vi "main -2.0.vi"() -> ()   [LabVIEW 2018]
uses:
  <vilib>/Analysis/baseanly.llb/Mean (DBL).vi
  <vilib>/Instr/_visa.llb/VISA Configure Serial Port (Instr).vi
  <vilib>/Analysis/NI_AALBase.lvlib
panel:
  out "十六进制整型字符串":string
  out "提示":string
  out "错误指示":bool
  in  "单片机COM":refnum<visa-resource-name>
  out "上一路数据图":dbl[](graph)
  in  "数据存储位置":path
  in  "开关":bool
  out "2-7 2":bool
  out "2-6 2":bool
  out "2-5 2":bool
  out "2-4 2":bool
  out "2-3 2":bool
  out "2-2 2":bool
  out "2-1 2":bool
  out "1-7 2":bool
  out "1-6 2":bool
  out "1-5 2":bool
  out "1-4 2":bool
  out "1-3 2":bool
  out "1-2 2":bool
  out "1-1 2":bool
  out "字符串":string
  in  "1-7":bool
  in  "2-7":bool
  in  "2-6":bool
  in  "2-5":bool
  in  "2-4":bool
  in  "2-3":bool
  in  "2-2":bool
  in  "2-1":bool
  in  "1-1":bool
  in  "1-2":bool
  in  "1-3":bool
  in  "1-4":bool
  in  "1-5":bool
  in  "1-6":bool
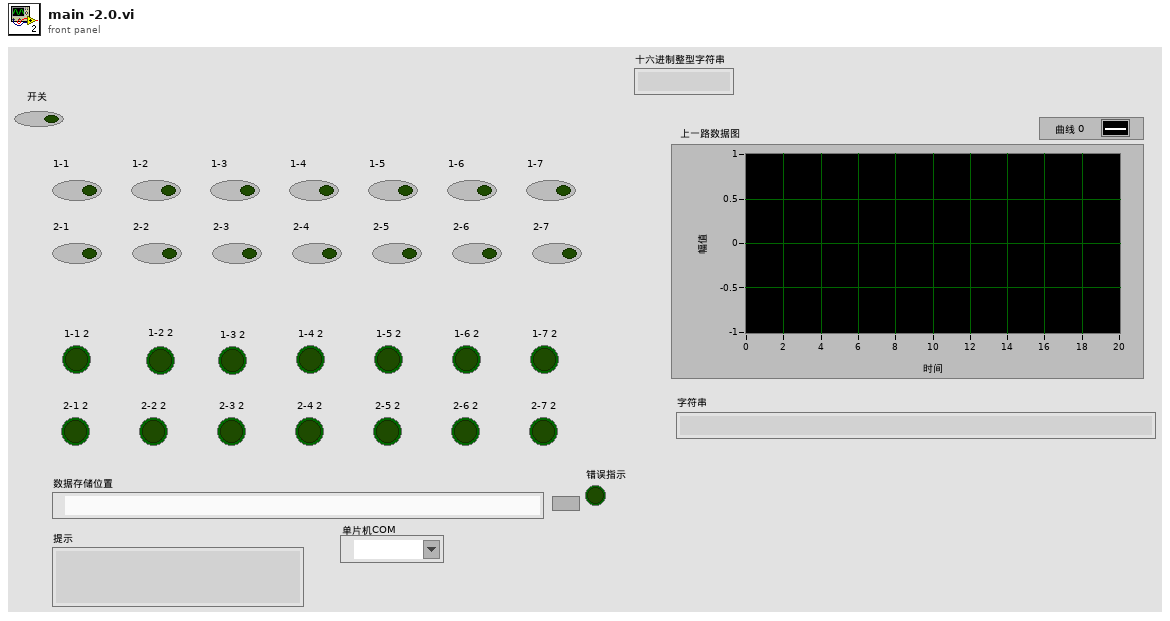
[diagram p1: front panel]
types:
  T1 = enum16{"open", "replace", "create", "open or create", "replace or create", "replace or create with confirmation"}
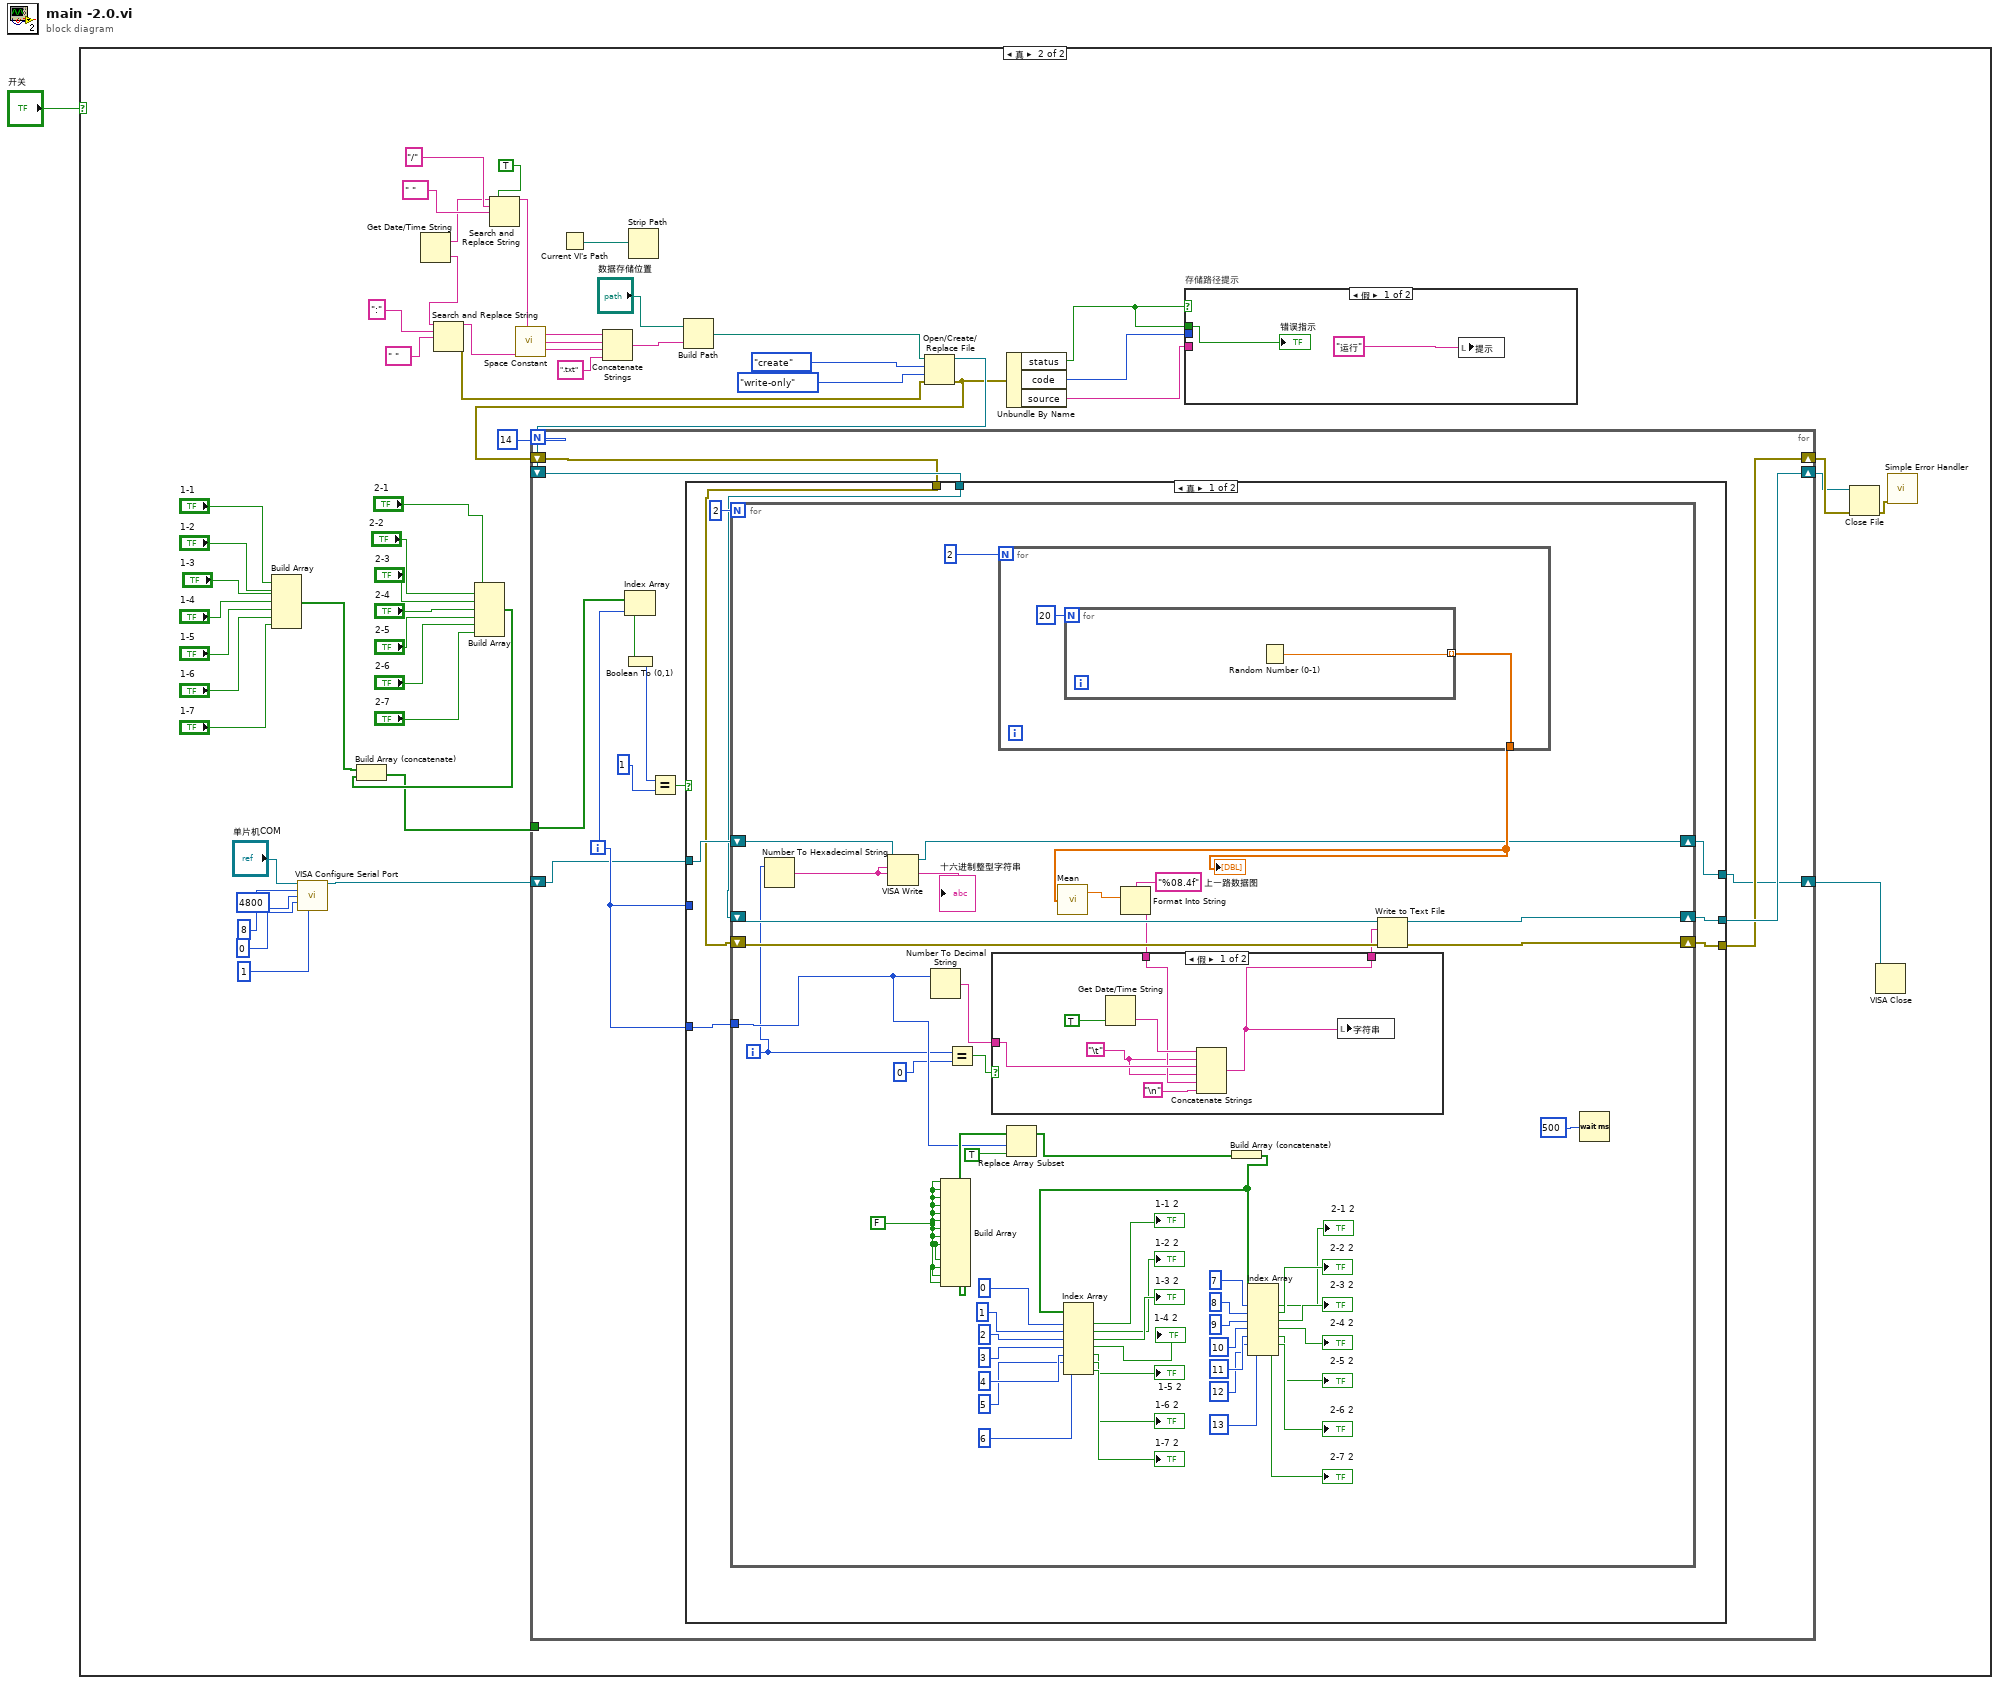
[diagram p0: block diagram]
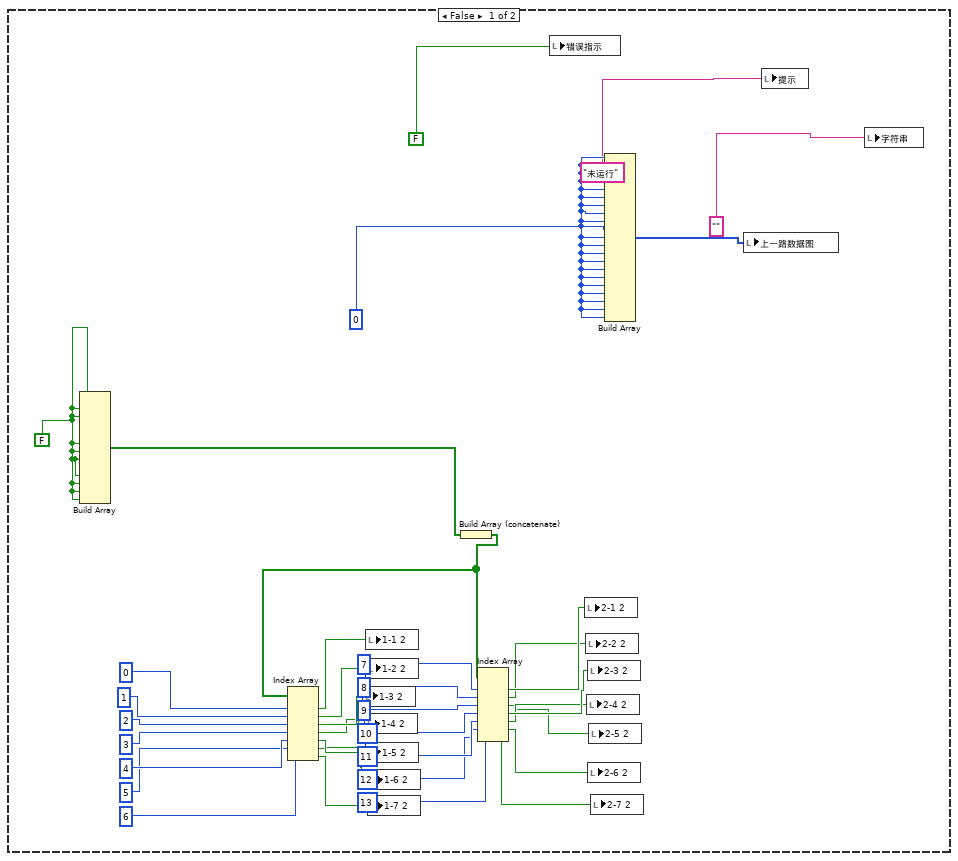
[diagram p2: hidden frame]
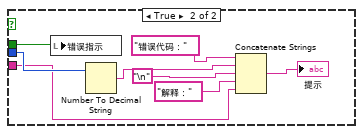
[diagram p3: hidden frame]
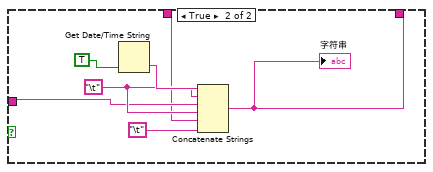
[diagram p4: hidden frame]
diagram:
  n1 = case shown="真" "开关" {
    frame False {
      w5 = 0
      w37 = FALSE
      n2 = Build Array(w37, w37, w37, w37, w37, w37, w37, w37, w37, w37, w37, w37, w37, w37) -> (w21:bool[])
      n3 = Build Array (concatenate)(w21) -> (w36:bool[])
      n4 = Index Array(array=w36, index #1=0, index #2=1, index #3=2, index #4=3, index #5=4, index #6=5, index #7=6) -> (element #1=w13:bool, element #2=w12:bool, element #3=w11:bool, element #4=w10:bool, element #5=w9:bool, element #6=w8:bool, element #7=w7:bool)
      n5 = local write "1-3 2"(w11) -> ()
      n6 = local write "1-4 2"(w10) -> ()
      n7 = local write "1-1 2"(w13) -> ()
      n8 = local write "1-2 2"(w12) -> ()
      n9 = local write "1-5 2"(w9) -> ()
      n10 = local write "1-6 2"(w8) -> ()
      n11 = local write "1-7 2"(w7) -> ()
      n12 = Index Array(array=w36, index #1=7, index #2=8, index #3=9, index #4=10, index #5=11, index #6=12, index #7=13) -> (element #1=w20:bool, element #2=w19:bool, element #3=w16:bool, element #4=w18:bool, element #5=w17:bool, element #6=w15:bool, element #7=w14:bool)
      n13 = local write "错误指示"(FALSE) -> ()
      n14 = local write "2-1 2"(w20) -> ()
      n15 = local write "2-2 2"(w19) -> ()
      n16 = local write "2-4 2"(w17) -> ()
      n17 = local write "2-3 2"(w18) -> ()
      n18 = local write "2-6 2"(w15) -> ()
      n19 = local write "2-5 2"(w16) -> ()
      n20 = local write "2-7 2"(w14) -> ()
      n21 = Build Array(w5, w5, w5, w5, w5, w5, w5, w5, w5, w5, w5, w5, w5, w5, w5, w5, w5, w5, w5, w5, w5) -> (w6:i32[])
      n22 = local write "上一路数据图"(w6) -> ()
      n23 = local write "提示"("未运行") -> ()
      n24 = local write "字符串"("") -> ()
    }
    frame True {
      n25 = Build Array("1-1", "1-2", "1-3", "1-4", "1-5", "1-6", "1-7") -> (w74:bool[])
      n26 = call-poly "VISA Configure Serial Port"("VISA resource name"="单片机COM", "baud rate (9600)"=4800, "data bits (8)"=8, "parity (0:none)"=0, "stop bits (10: 1 bit)"=1) -> ("VISA resource name out"=w42:refnum<visa-resource-name>)  [unwired: 9 in, 1 out]
      n27 = Get Date/Time String() -> (date string=w56:string, time string=w63:string)  [unwired: 3 in]
      n28 = Search and Replace String(input string=w63, search string=":", replace string=" ") -> (result string=w53:string, error out=w60:errorcluster)  [unwired: 5 in, 2 out]
      n29 = Build Array("2-1", "2-2", "2-3", "2-4", "2-5", "2-6", "2-7") -> (w73:bool[])
      n30 = Build Array (concatenate)(w74, w73) -> (w72:bool[])
      n31 = Search and Replace String(replace all?=TRUE, input string=w56, search string="/", replace string=" ") -> (result string=w55:string)  [unwired: 4 in, 3 out]
      n32 = call <vilib>:"Space Constant.vi"() -> ("String"=w59:string)
      n33 = Current VI's Path() -> (path=w66:path)
      n34 = Concatenate Strings(w55, w59, w53, ".txt") -> (w70:string)
      n35 = Strip Path(path=w66) -> ()  [unwired: 2 out]
      n36 = Build Path(base path="数据存储位置", name or relative path=w70) -> (appended path=w65:path)
      n37 = Open/Create/Replace File(file path (use dialog)=w65, error in=w60, operation (0:open)=T1."create", access (0:read/write)=enum16{"read/write", "read-only", "write-only"}."write-only") -> (refnum out=w67:refnum<file>, error out=w41:errorcluster)  [unwired: 3 out]
      n38 = for {
        N: 14 -> [_]
        tunnel: w72 -> [w102]
        shift-right: [w106] -> w51
        shift-left: w67 -> [w104]
        shift-right: [w105] -> w52
        shift-left: w41 -> [w103]
        shift-right: [w99] -> w43
        shift-left: w42 -> [w100]
        i -> [w101]
        n39 = Index Array(array=w102, index=w101) -> (element=w110:bool)
        n40 = Boolean To (0,1)(Boolean=w110) -> (0, 1=w108:i16)
        n41 = Equal?(x=w108, y=1) -> (x = y?=w107:bool)
        n42 = case shown="真" w107 {
          tunnel: w104 -> [w111 w189]
          tunnel: w101 -> [w116 _]
          tunnel: [w118 w189] -> w106
          tunnel: [w117 w190] -> w105
          tunnel: w103 -> [w112 w190]
          tunnel: w100 -> [w114 w188]
          tunnel: w101 -> [_ _]
          tunnel: [w113 w188] -> w99
          frame True {
            n43 = for {
              N: 2 -> [_]
              tunnel: w116 -> [w126]
              shift-right: [w169] -> w118
              shift-left: w111 -> [w170]
              shift-right: [w132] -> w117
              shift-left: w112 -> [w168]
              shift-right: [w121] -> w113
              shift-left: w114 -> [w122]
              i -> [w120]
              w165 = FALSE
              n44 = Number To Hexadecimal String(2:w120) -> (0:w119:string)  [unwired: 1 in]
              "十六进制整型字符串" <- w119
              n45 = VISA Write(VISA resource name=w122, write buffer=w119) -> (VISA resource name out=w121:refnum<visa-resource-name>)  [unwired: 1 in, 2 out]
              n46 = Number To Decimal String(number=w126) -> (decimal integer string=w167:string)  [unwired: 1 in]
              n47 = Build Array(w165, w165, w165, w165, w165, w165, w165, w165, w165, w165, w165, w165, w165, w165) -> (w164:bool[])
              n48 = Equal?(x=w120, y=0) -> (x = y?=w124:bool)
              n49 = for {
                N: 2 -> [_]
                tunnel: [w186] -> w128
                n50 = for {
                  N: 20 -> [_]
                  tunnel: [w187] -> w186 mode=indexing
                  n51 = Random Number (0-1)() -> (number: 0 to 1=w187:dbl)
                }
              }
              "上一路数据图" <- w128
              n52 = Replace Array Subset(array=w164, new element=TRUE, index=w126) -> (w133:bool[])
              n53 = call-poly <vilib>:"Mean.vi"("X"=w128) -> ("mean"=w130:dbl)  [unwired: 1 out]
              n54 = Format Into String(format string="%08.4f" ("格式字符串"), w130) -> (resulting string=w129:string)  [unwired: 2 in, 1 out]
              n55 = case shown="假" w124 {
                tunnel: w167 -> [w174 w181]
                tunnel: [w171 w180] -> w166
                tunnel: w129 -> [w173 w179]
                frame False {
                  w172 = "\t" ("Tab")
                  n56 = Get Date/Time String(want seconds? (F)=TRUE) -> (time string=w176:string)  [unwired: 2 in, 1 out]
                  n57 = Concatenate Strings(w176, w172, w174, w172, w173, "\n") -> (w171:string)
                  n58 = local write "字符串"(w171) -> ()
                }
                frame True {
                  w182 = "\t" ("Tab")
                  n59 = Get Date/Time String(want seconds? (F)=TRUE) -> (time string=w183:string)  [unwired: 2 in, 1 out]
                  n60 = Concatenate Strings(w183, w182, w181, w182, w179, "\t") -> (w180:string)
                  "字符串" <- w180
                }
              }
              n61 = Build Array (concatenate)(w133) -> (w148:bool[])
              n62 = Index Array(array=w148, index #1=0, index #2=1, index #3=2, index #4=3, index #5=4, index #6=5, index #7=6) -> (element #1=→"1-1 2":bool, element #2=→"1-2 2":bool, element #3=→"1-3 2":bool, element #4=→"1-4 2":bool, element #5=→"1-5 2":bool, element #6=→"1-6 2":bool, element #7=→"1-7 2":bool)
              n63 = Index Array(array=w148, index #1=7, index #2=8, index #3=9, index #4=10, index #5=11, index #6=12, index #7=13) -> (element #1=→"2-1 2":bool, element #2=→"2-2 2":bool, element #3=→"2-3 2":bool, element #4=→"2-4 2":bool, element #5=→"2-5 2":bool, element #6=→"2-6 2":bool, element #7=→"2-7 2":bool)
              n64 = Write to Text File(file (use dialog)=w170, text=w166, error in=w168) -> (refnum out=w169:refnum<file>, error out=w132:errorcluster)  [unwired: 1 in, 1 out]
              n65 = Wait (ms)(milliseconds to wait=u32 500) -> ()  [unwired: 1 out]
            }
          }
          frame False {
          }
        }
      }
      n66 = Unbundle By Name(w41) -> ("status"=w38:bool, "code"=w40:i32, "source"=w39:string)
      n67 = case "存储路径提示" shown="假" w38 {
        tunnel: w40 -> [_ w97]
        tunnel: w39 -> [_ w92]
        tunnel: w38 -> [w90 w98]
        frame False {
          n68 = local write "提示"("运行") -> ()
          "错误指示" <- w90
        }
        frame True {
          n69 = local write "错误指示"(w98) -> ()
          n70 = Number To Decimal String(number=w97) -> (decimal integer string=w95:string)  [unwired: 1 in]
          n71 = Concatenate Strings("错误代码：", w95, "\n", "解释：", w92) -> (→"提示":string)
        }
      }
      n72 = Close File(refnum=w51, error in=w52) -> (error out=w50:errorcluster)  [unwired: 1 out]
      n73 = VISA Close(VISA resource name=w43) -> ()  [unwired: 1 in, 1 out]
      n74 = call <vilib>:"Simple Error Handler.vi"("error in (no error)"=w50) -> ()  [unwired: 2 in, 7 out]
    }
  }
